vi "FanSimulation.vi"() -> ()   [LabVIEW 2021]
panel:
  in  "Speed'":dbl(knob)
  in  "Stop":bool
  out "Ring":u16(ring)
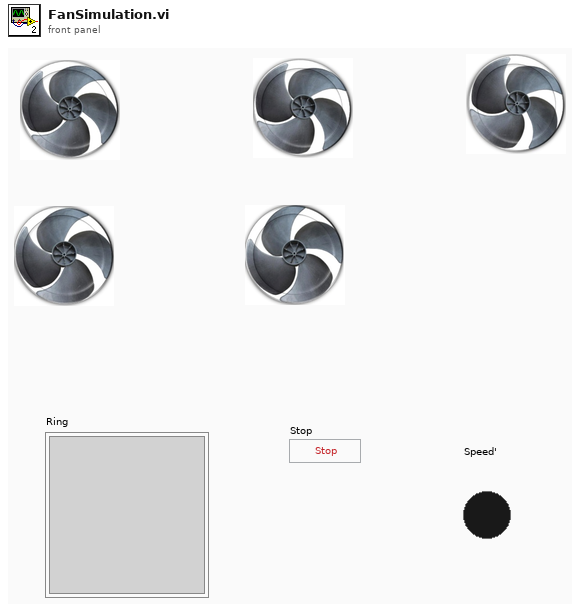
[diagram p1: front panel]
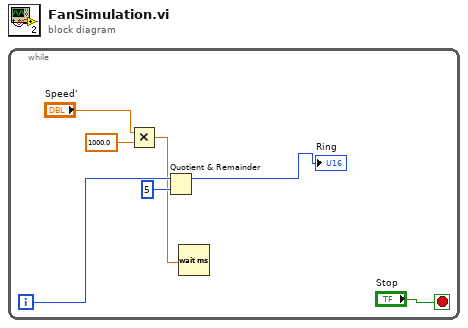
[diagram p0: block diagram]
diagram:
  n1 = while {
    i -> [w6]
    stop <- "Stop" stop-if-true
    n2 = Multiply(x="Speed'", y=1000.0) -> (x*y=w1:dbl)
    n3 = Quotient & Remainder(x=w6, y=5) -> (x-y*floor(x/y)=→"Ring":i32)  [unwired: 1 out]
    n4 = Wait (ms)(milliseconds to wait=w1) -> ()  [unwired: 1 out]
  }
